vi "StatusChange.vi"(8 "error in (no error)":errorcluster, 11 "MGI_MenuItem in":refnum<class "MGI_MenuItem.lvclass">) -> (0 "error out":errorcluster, 3 "MGI_MenuItem out":refnum<class "MGI_MenuItem.lvclass">)   [LabVIEW 2016, in "MGI_MenuItem.lvclass"]
doc: "Generates the user event to indicate the status of the menu item has changed.\n\nAuthored by Derek E. Trepanier\nsupport@mooregoodideas.com\nwww.mooregoodideas.com\n\nCopyright (c) 2012, Moore Good Ideas, Inc.\n\nAll rights reserved.\n\nRedistribution and use in source and binary forms, with or without modification, are permitted provided that the following conditions are met:\n\n * Redistributions of source code must retain the above copyright notice, this list of conditions and the following disclaimer.\n * Redistributions in binary form must reproduce the above copyright notice, this list of conditions and the following disclaimer in the documentation and/or other materials provided with the distribution.\n * Neither the name of Moore Good Ideas, Inc. nor the names of its contributors may be used to endorse or promote products derived from this software without specific prior written permission.\n\nTHIS SOFTWARE IS PROVIDED BY THE COPYRIGHT HOLDERS AND CONTRIBUTORS \"AS IS\" AND ANY EXPRESS OR IMPLIED WARRANTIES, INCLUDING, BUT NOT LIMITED TO, THE IMPLIED WARRANTIES OF MERCHANTABILITY AND FITNESS FOR A PARTICULAR PURPOSE ARE DISCLAIMED. IN NO EVENT SHALL THE COPYRIGHT OWNER OR CONTRIBUTORS BE LIABLE FOR ANY DIRECT, INDIRECT, INCIDENTAL, SPECIAL, EXEMPLARY, OR CONSEQUENTIAL DAMAGES (INCLUDING, BUT NOT LIMITED TO, PROCUREMENT OF SUBSTITUTE GOODS OR SERVICES; LOSS OF USE, DATA, OR PROFITS; OR BUSINESS INTERRUPTION) HOWEVER CAUSED AND ON ANY THEORY OF LIABILITY, WHETHER IN CONTRACT, STRICT LIABILITY, OR TORT (INCLUDING NEGLIGENCE OR OTHERWISE) ARISING IN ANY WAY OUT OF THE USE OF THIS SOFTWARE, EVEN IF ADVISED OF THE POSSIBILITY OF SUCH DAMAGE."
uses:
  <userlib>/_MGI/Menu Building/MenuItem/MGI_MenuItem.lvclass
  <userlib>/_MGI/Menu Building/MenuItem/MGI_MenuItem.lvclass/MGI_MenuItem.ctl
  <userlib>/_MGI/Menu Building/MenuItemStatusChange/MGI_MenuItemStatusChange.lvclass
  <userlib>/_MGI/Menu Building/MenuTypes/MGI_Menu.lvclass
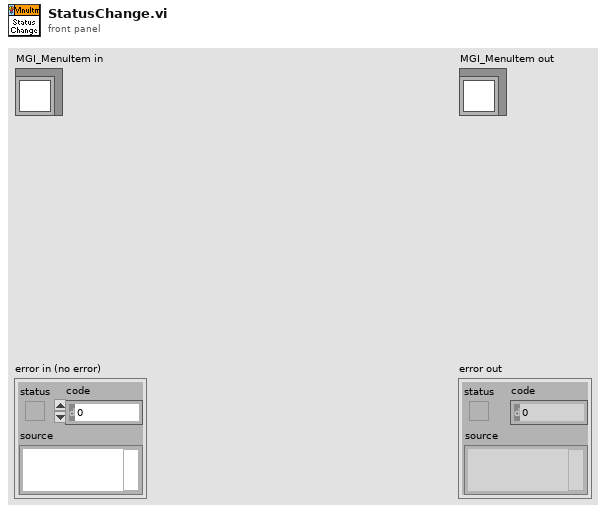
[diagram p1: front panel]
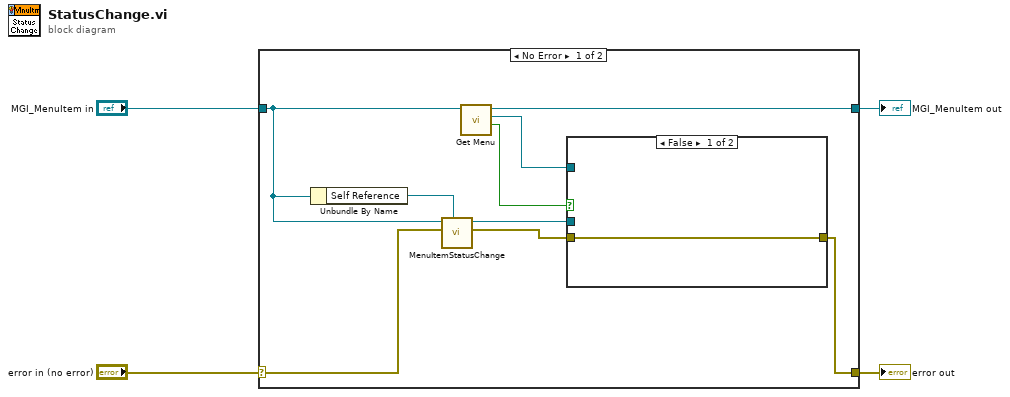
[diagram p0: block diagram]
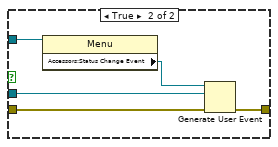
[diagram p2: hidden frame]
diagram:
  n1 = case shown="No Error" "error in (no error)" {
    selector: "error in (no error)" -> [w5 w21]
    tunnel: [w13 w21] -> w3
    tunnel: [w11 w20] -> w1
    tunnel: "MGI_MenuItem in" -> [w6 w20]
    frame No Error {
      n2 = Unbundle By Name(w6) -> ("Self Reference"=w7:refnum<data-value>)
      n3 = call <userlib>:"MenuItemStatusChange.vi"("MenuItem"=w7, "error in (no error)"=w5, "MenuItem before Click"=w6) -> ("error out"=w8:errorcluster, "MenuItemStatusChange out"=w9:refnum<class "MGI_MenuItemStatusChange.lvclass">)  [unwired: 7 in]
      n4 = call <userlib>:"Get Menu.vi"("MenuItem in"=w6) -> ("Menu Valid"=w10:bool, "Menu"=w12:refnum<class "MGI_Menu.lvclass">, "MenuItem out"=w11:refnum<class "MGI_MenuItem.lvclass">)  [unwired: 7 in, 1 out]
      n5 = case shown="False" w10 {
        tunnel: [w14 w19] -> w13
        tunnel: w8 -> [w14 w18]
        tunnel: w9 -> [_ w16]
        tunnel: w12 -> [_ w15]
        frame False {
        }
        frame True {
          n6 = property class="Menu"(reference=w15) -> ("Accessors:Status Change Event"=w17:refnum<user-event>)  [unwired: 1 in, 2 out]
          n7 = Generate User Event(user event=w17, event data cluster=w16, error in=w18) -> (error out=w19:errorcluster)  [unwired: 1 in, 1 out]
        }
      }
    }
    frame Error {
    }
  }
  "error out" <- w3
  "MGI_MenuItem out" <- w1
